vi "VarToData - TimeSeries.vi"(4 "error in":errorcluster, 6 "data":variant) -> (0 "error out":errorcluster, 1 "TSFrames":i32, 2 "Exp params":T1={"Experiment Type"="Dynamic Time Series", "Experiment Name"="Experiment_1", "ExpPath"=path "D:/Data", "Save As"="TIFF", "TSFrames"=1000, "TSfps"=1.0, "Streaming"=FALSE, "tdms ref"=refnum, "frame #"=0, "Full Path"=path "", "PeakOnQueue"=FALSE} {"TSFrames" min=1 step=1; "TSfps" min=0.001 max=90.0 step=0.001 format="%_4g"})   [LabVIEW 2020]
uses:
  _controls/Exp Params.ctl
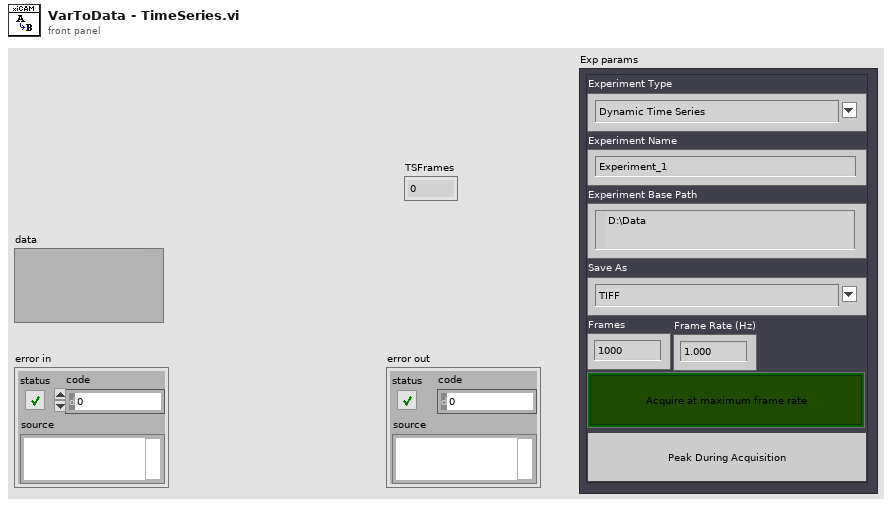
[diagram p1: front panel]
types:
  T1 = typedef "Exp Params.ctl" = cluster{"Experiment Type":string, "Experiment Name":string, "ExpPath":path, "Save As":string, "TSFrames":i32, "TSfps":dbl, "Streaming":bool, "tdms ref":refnum<k34>, "frame #":i64, "Full Path":path, "PeakOnQueue":bool}
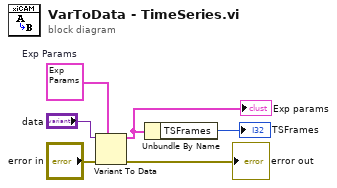
[diagram p0: block diagram]
diagram:
  w4 = T1 {"Experiment Type"="", "Experiment Name"="", "ExpPath"=path "", "Save As"="", "TSFrames"=0, "TSfps"=0.0, "Streaming"=FALSE, "tdms ref"=refnum, "frame #"=0, "Full Path"=path "", "PeakOnQueue"=FALSE}  # Exp Params
  n1 = Variant To Data(error in="error in", type=w4, Variant="data") -> (data=w6:T1, error out=→"error out":errorcluster)
  "Exp params" <- w6
  n2 = Unbundle By Name(w6) -> ("TSFrames"=→"TSFrames":i32)
